vi "Output.vi"(8 "error in (no error)":errorcluster, 11 "PID in":refnum<class "PID.lvclass">) -> (0 "error out":errorcluster, 2 "Output":dbl, 3 "PID out":refnum<class "PID.lvclass">)   [LabVIEW 2024, in "PID.lvlib" / "PID.lvclass"]
uses:
  PID.lvclass
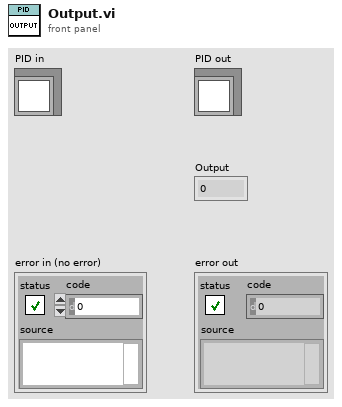
[diagram p1: front panel]
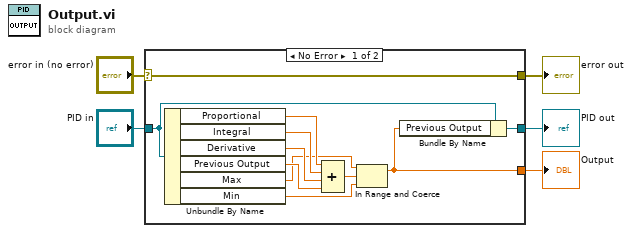
[diagram p0: block diagram]
diagram:
  n1 = case shown="No Error" "error in (no error)" {
    selector: "error in (no error)" -> [w16 w18]
    tunnel: [w16 w18] -> w4
    tunnel: [w6 w17] -> w2
    tunnel: "PID in" -> [w8 w17]
    tunnel: [w7 _] -> w1
    frame No Error {
      n2 = Unbundle By Name(w8) -> ("Proportional"=w15:dbl, "Integral"=w14:dbl, "Derivative"=w13:dbl, "Previous Output"=w12:dbl, "Max"=w10:dbl, "Min"=w9:dbl)
      n3 = Compound Arithmetic op=ADD(w15, w14, w13, w12) -> (w11:dbl)
      n4 = In Range and Coerce(upper limit=w10, x=w11, lower limit=w9) -> (coerced(x)=w7:dbl)  [unwired: 1 out]
      n5 = Bundle By Name(cluster=w8, "Previous Output"=w7) -> (w6:refnum<class "PID.lvclass">)
    }
    frame Error {
    }
  }
  "error out" <- w4
  "PID out" <- w2
  "Output" <- w1
